vi "Synth Program Outputs.vi"(2 "Match clocks":bool=TRUE, 4 "Use hardware clock for DO":bool, 5 "Mode":T3(ring), 6 "IF (Hz)":dbl=1000.0, 7 "Phase (degrees)":dbl min=0.0 max=360.0 step=11.25, 8 "error in (no error)":errorcluster, 9 "Clock Multiplier":i32=64, 10 "DAQmx Device Name":tag="6251", 11 "f (Hz)":dbl) -> (0 "error out":errorcluster, 1 "Lockin parameters array":T1[](array[typedef]) {"DDS clock" format="%_17pHz"; "DDS modulus" format="0x%x (%d)"; "Phase" format="%#_gdeg"; "Frequency" format="%_17pHz"}, 3 "Actual ratios":T2 {"Clock" format="%_20p"; "F2" format="%_20p"; "F1" format="%_20p"; "Clock/F2" format="%_20g"; "Clock/F1" format="%_20g"})   [LabVIEW 2016]
uses:
  Actual Settings.ctl
  SoftwareLockin/Lockin Parameters.ctl
  <vilib>/DAQmx/write.llb/DAQmx Write (Digital 1D U8 1Chan NSamp).vi
  <vilib>/DAQmx/miscellaneous.llb/DAQmx Fill In Error Info.vi
panel:
  out "Variable F-word":u32
  out "Fixed F-word":u32
  out "Clock F-word":u32
  out "Full Byte Array":u8[](array[numeric]) format="%08b"
  in  "Delay (ms)":u32=1
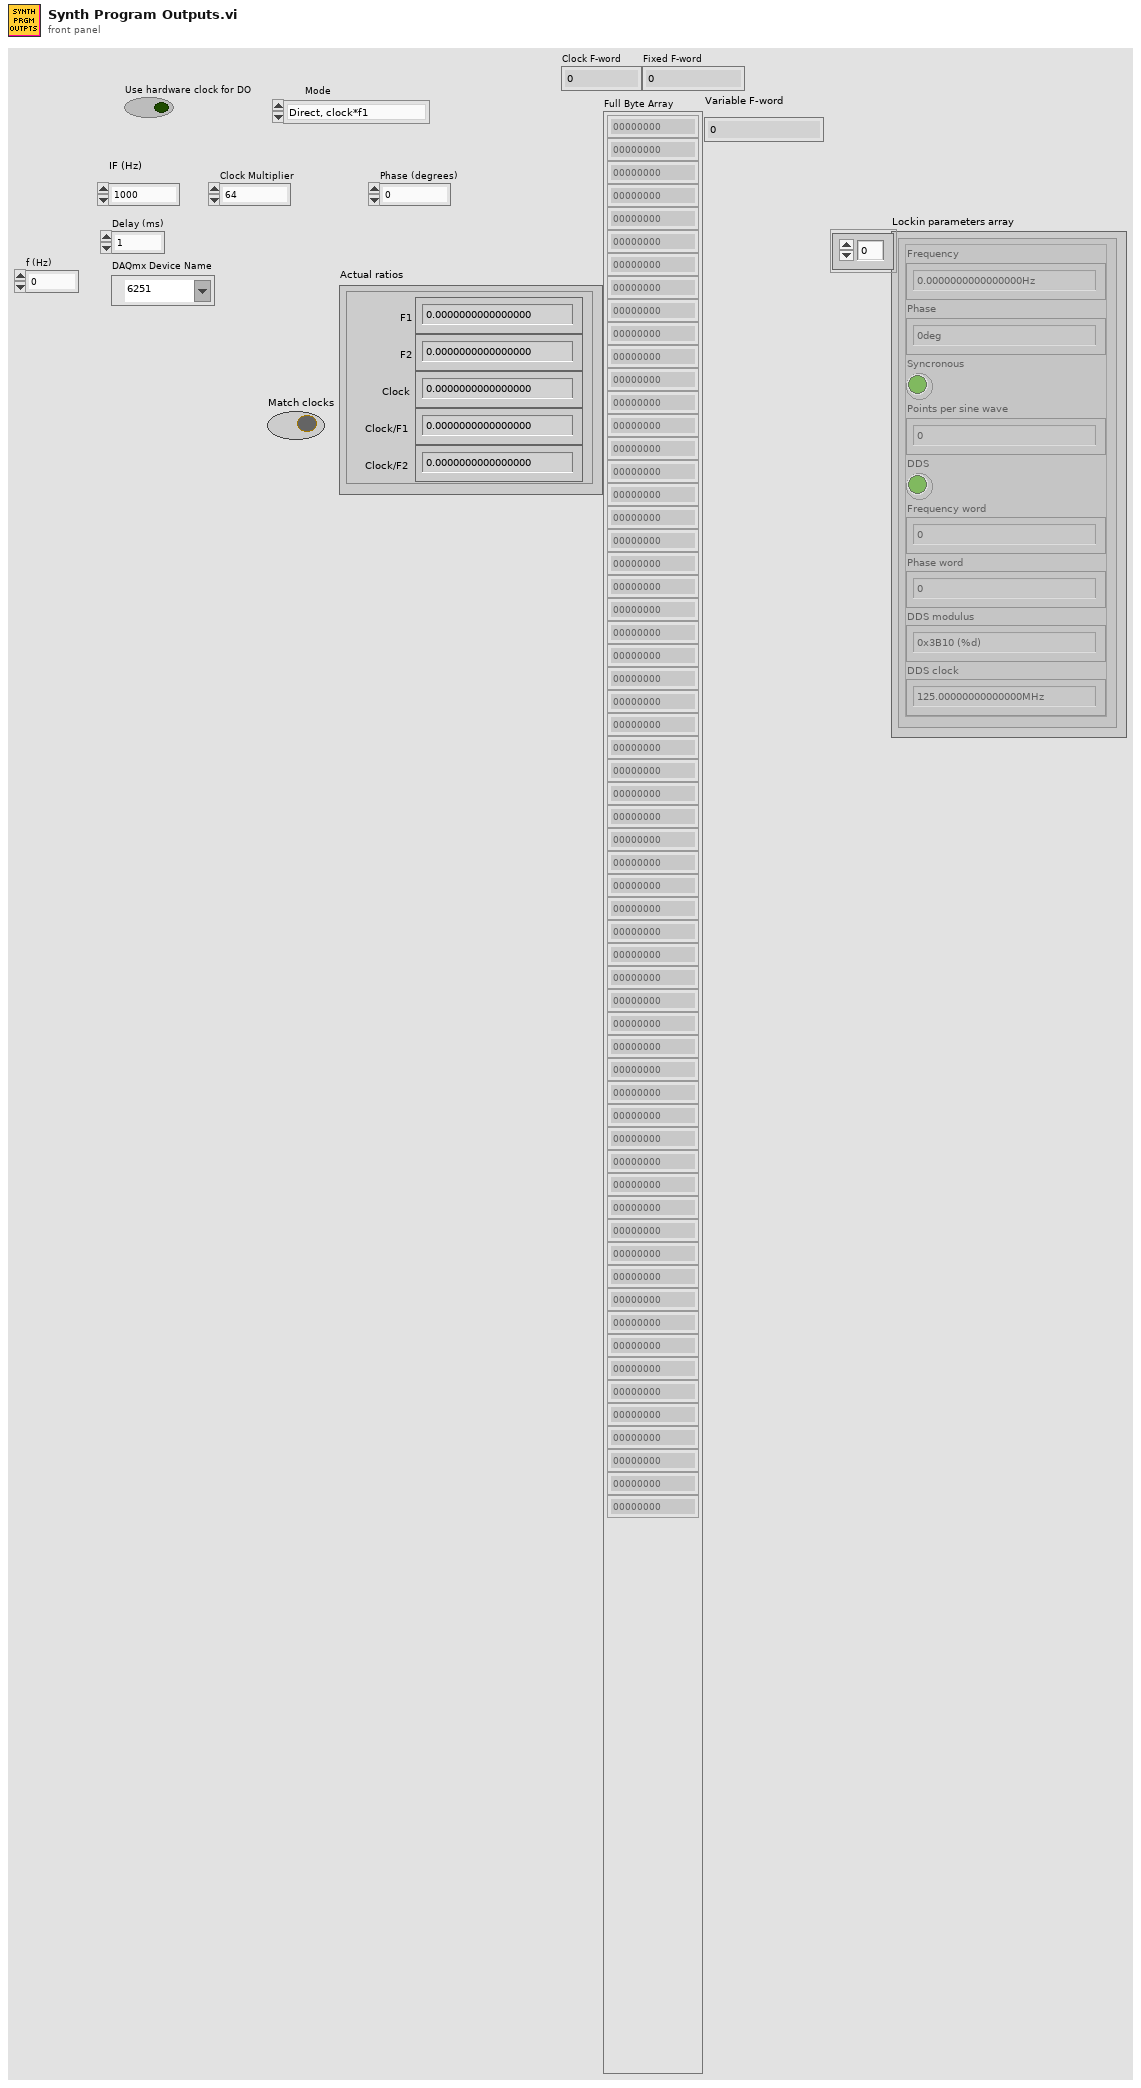
[diagram p1: front panel]
types:
  T1 = typedef "Lockin Parameters.ctl" = cluster{"Frequency":dbl, "Phase":dbl, "Syncronous":bool, "Points per sine wave":i32, "DDS":bool, "Frequency word":u32, "Phase word":u32, "DDS modulus":i64, "DDS clock":dbl}
  T2 = typedef "Actual settings.ctl" = cluster{"Clock/F1":ext, "Clock/F2":ext, "F1":ext, "F2":ext, "Clock":ext}
  T3 = enum16{"Direct, clock*f1", "Direct, clock*f2", "Heterodyne"}
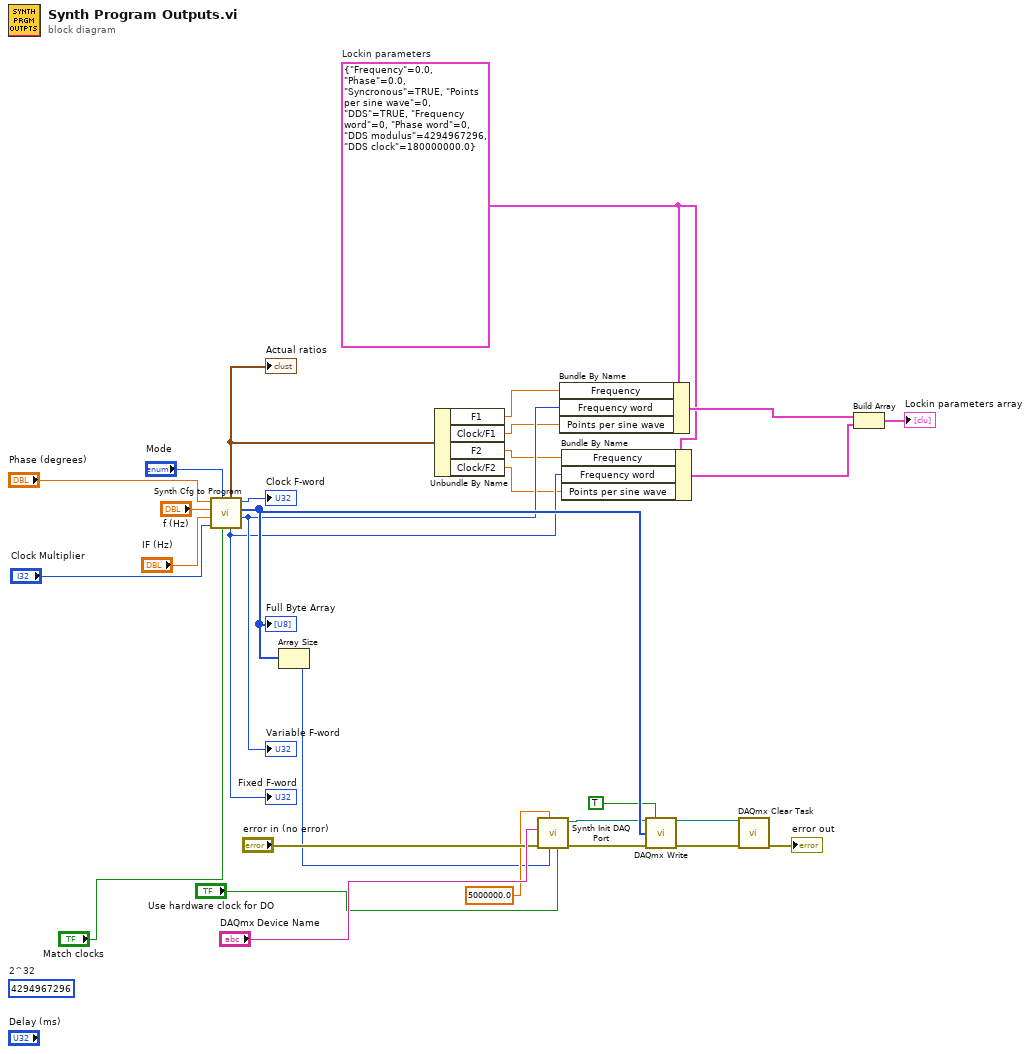
[diagram p0: block diagram]
diagram:
  (unwired) u64 4294967296  # 2^32
  w3 = T1 {"Frequency"=0.0, "Phase"=0.0, "Syncronous"=TRUE, "Points per sine wave"=0, "DDS"=TRUE, "Frequency word"=0, "Phase word"=0, "DDS modulus"=4294967296, "DDS clock"=180000000.0}  # Lockin parameters
  n1 = call "Synth Cfg to Program.vi"("Match clocks"="Match clocks", "Mode"="Mode", "Clock Multiplier"="Clock Multiplier", "IF (Hz)"="IF (Hz)", "f (Hz)"="f (Hz)", "Phase (degrees)"="Phase (degrees)") -> ("f"=w11:u32, "Full Byte Array"=w19:u8[], "Clock F-word"=→"Clock F-word":u32, "Fixed F-word"=w7:u32, "Actual ratios"=w10:T2)  [unwired: 1 out]
  "Full Byte Array" <- w19
  "Actual ratios" <- w10
  "Fixed F-word" <- w7
  "Variable F-word" <- w11
  n2 = Array Size(array=w19) -> (size(s)=w21:i32)
  n3 = Unbundle By Name(w10) -> ("F1"=w9:ext, "Clock/F1"=w6:ext, "F2"=w8:ext, "Clock/F2"=w5:ext)
  n4 = call "Synth Init DAQ Port.vi"("Use hardware clock for DO"="Use hardware clock for DO", "DO Samples per Channel"=w21, "DO Clock Rate (Hz)"=5000000.0 ("Sample Clock Rate (Hz)"), "error in (no error)"="error in (no error)", "DAQmx Device Name"="DAQmx Device Name") -> ("error out"=w16:errorcluster, "task out"=w15:refnum<k21>)  [unwired: 5 in]
  n5 = Bundle By Name(cluster=w3, "Frequency"=w9, "Frequency word"=w11, "Points per sine wave"=w6) -> (w4:T1)
  n6 = Bundle By Name(cluster=w3, "Frequency"=w8, "Frequency word"=w7, "Points per sine wave"=w5) -> (w2:T1)
  n7 = call-poly <vilib>:"DAQmx Write.vi"("task/channels in"=w15, "auto start"=TRUE, "data"=w19, "error in"=w16) -> ("task out"=w17:refnum<k21>, "error out"=w18:errorcluster)  [unwired: 9 in, 1 out]
  n8 = call <vilib>:"DAQmx Clear Task.vi"("task in"=w17, "error in"=w18) -> ("error out"=→"error out":errorcluster)  [unwired: 13 out]
  n9 = Build Array(w4, w2) -> (→"Lockin parameters array":T1[])
